vi "Test Coffee Shop Add Cashier Broadcast Name.vi"(8 "error in (no error)":errorcluster, 11 "Coffee Shop Test In":refnum<class "Coffee Shop Test.lvclass">) -> (0 "error out":errorcluster, 3 "Coffee Shop Test Out":refnum<class "Coffee Shop Test.lvclass">)   [LabVIEW 2020, in "Coffee Shop Test.lvclass"]
uses:
  Coffee Shop Test.lvclass
  C:/Program Files (x86)/National Instruments/LabVIEW 2020/vi.lib/Astemes/LUnit/Test Case.lvclass
  Processes/Coffee Shop/Coffee Shop.lvclass
  C:/Program Files (x86)/National Instruments/LabVIEW 2020/vi.lib/Astemes/Triarc Framework/Process/Process.lvclass
  <vilib>/Astemes/Triarc Framework/Process/Process.lvclass/Process.ctl
  <vilib>/Astemes/LUnit/Test Case.lvclass/Test Case.ctl
  1b512e5e-f5c2-4463-8958-f8337bec37b2.vi
  <vilib>/Astemes/Triarc Framework/Process/Public/Lifecycle/Get Lifecycle State.vi
  <vilib>/Astemes/Triarc Framework/Support/Execution timer.vi
  <vilib>/Astemes/Triarc Framework/Process/Private/SubVIs/Wait for finish.vi
  <vilib>/Astemes/Triarc Framework/Process/Private/SubVIs/Set Lifecycle State.vi
  <vilib>/Astemes/Triarc Framework/Process/Protected/Messaging/Send Message.vi
  <vilib>/Astemes/LUnit/Append Pass Result.vi
  <vilib>/Astemes/LUnit/Append Fail Result.vi
  <vilib>/Astemes/LUnit/Describe Comparison.vi
  <vilib>/Astemes/LUnit/Compare Variants.vi
  <vilib>/Utility/error.llb/Clear Errors.vi
  <vilib>/Astemes/Triarc Framework/Process/Private/SubVIs/Handle Debug Data.vi
  <vilib>/Astemes/LUnit/Variant to string.vi
  <vilib>/Astemes/Triarc Framework/Logging/Log Debug.vi
  <vilib>/AdvancedString/1D String Array to Delimited String.vi
  <vilib>/Utility/High Resolution Relative Seconds.vi
  <vilib>/Utility/error.llb/Error Cluster From Error Code.vi
  <vilib>/Astemes/Triarc Framework/Support/Dequeue Broadcast Message.vi
  <vilib>/Astemes/Triarc Framework/Process/Public/Read Name.vi
  <vilib>/Utility/Data Type/Get Type Information.vi
  <vilib>/Utility/LVClass/Get LV Class Name.vi
  <vilib>/Astemes/Triarc Framework/Callback/Callback.lvclass
  <vilib>/Astemes/Triarc Framework/Process/Process.lvclass
  <vilib>/Astemes/Triarc Framework/Support/Broadcast Event Dequeuers.lvlib
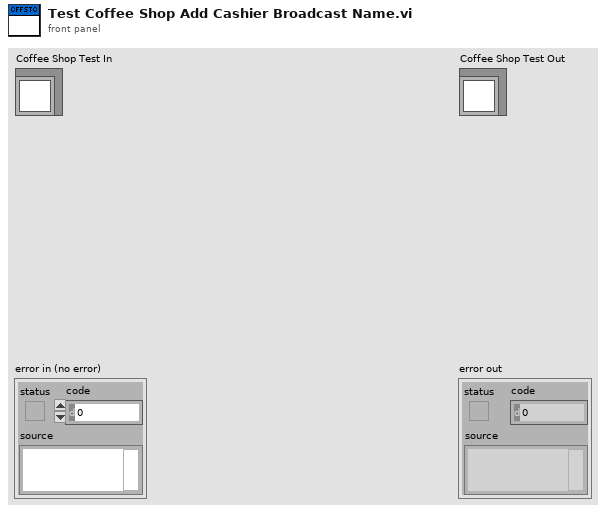
[diagram p1: front panel]
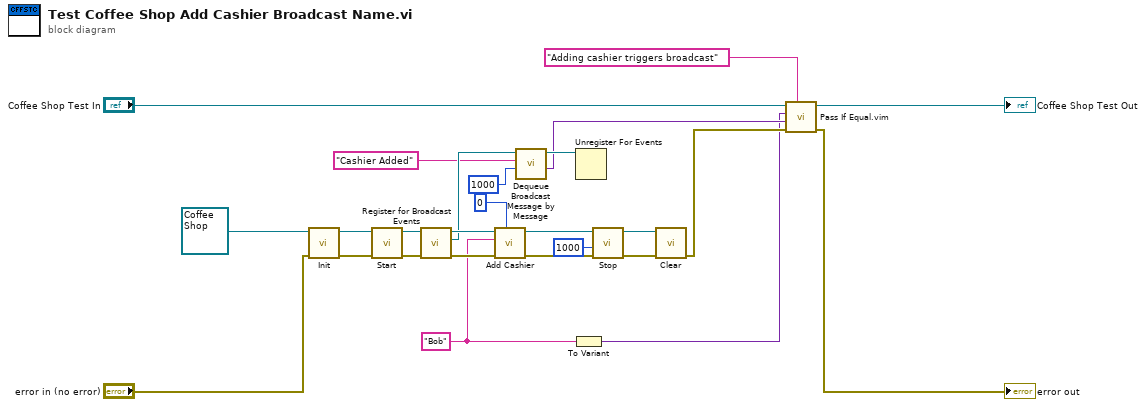
[diagram p0: block diagram]
diagram:
  w4 = "Bob" ("Name")
  n1 = call-dynamic "Init.vi"("error in (no error)"="error in (no error)", "Process In"=refnum<class "Coffee Shop.lvclass"> refnum ("Coffee Shop.lvclass")) -> ("error out"=w24:errorcluster, "Process Out"=w25:refnum<class "Coffee Shop.lvclass">)  [unwired: 8 in]
  n2 = call <vilib>:"Start.vi"("error in (no error)"=w24, "Process In"=w25) -> ("error out"=w23:errorcluster, "Process Out"=w16:refnum<class "Coffee Shop.lvclass">)  [unwired: 7 in, 1 out]
  n3 = call <vilib>:"Register for Broadcast Events.vi"("error in (no error)"=w23, "Process In"=w16) -> ("error out"=w17:errorcluster, "Event Registration Refnum Out"=w14:refnum<event-registration>, "Process Out"=w15:refnum<class "Coffee Shop.lvclass">)  [unwired: 7 in]
  n4 = call "Add Cashier.vi"("Time Scale [ms]"=u32 0, "error in (no error)"=w17, "Name"=w4, "Coffee Shop in"=w15) -> ("error out"=w19:errorcluster, "Coffee Shop out"=w18:refnum<class "Coffee Shop.lvclass">)  [unwired: 6 in]
  n5 = call <vilib>:"Dequeue Broadcast Message by Message.vi"("Timeout (-1)"=1000, "Message"="Cashier Added", "Event Registration Refnum"=w14) -> ("Message Data"=w5:variant, "Event Registration Refnum Out"=w12:refnum<event-registration>)  [unwired: 4 in, 3 out]
  n6 = To Variant(anything=w4) -> (Variant=w3:variant)
  n7 = Unregister For Events(event registration refnum=w12) -> ()  [unwired: 1 in, 1 out]
  n8 = call <vilib>:"Stop.vi"("error in (no error)"=w19, "timeout in ms (-1)"=1000, "Process In"=w18) -> ("error out"=w21:errorcluster, "Process Out"=w22:refnum<class "Coffee Shop.lvclass">)  [unwired: 6 in, 1 out]
  n9 = call-dynamic "Clear.vi"("error in (no error)"=w21, "Application In"=w22) -> ("error out"=w8:errorcluster)  [unwired: 9 in]
  n10 = call "Pass If Equal.vim"("Description"="Adding cashier triggers broadcast", "error in (no error)"=w8, "Actual"=w5, "Expected"=w3, "LUnit Test Case In"="Coffee Shop Test In") -> ("error out"=→"error out":errorcluster, "LUnit Test Case Out"=→"Coffee Shop Test Out":refnum<class "Coffee Shop Test.lvclass">)  [unwired: 5 in]
